vi "Check_Class_Spec.vi"(6 "ID String":string, 8 "error in (no error)":errorcluster, 9 "error out ref":refnum<vi>, 10 "vi refnum":refnum<vi>, 11 "ClassSpecifierConstant in":refnum<vi>) -> (0 "error out 2":errorcluster, 3 "OK":bool)   [LabVIEW 2025]
panel:
  out "error out":errorcluster
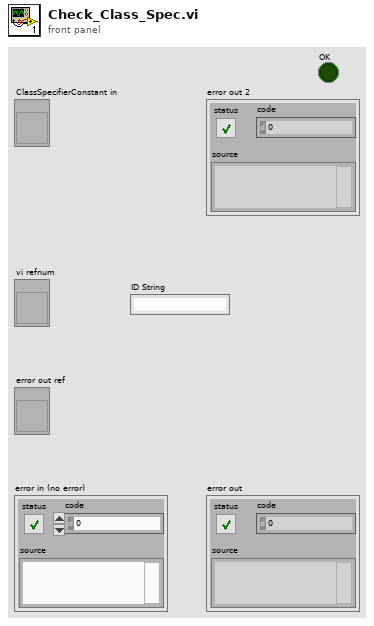
[diagram p1: front panel]
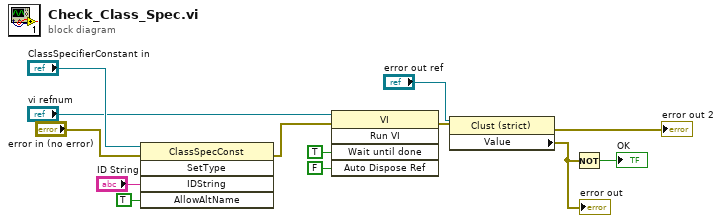
[diagram p0: block diagram]
diagram:
  n1 = invoke class="ClassSpecConst" method="SetType"(reference="ClassSpecifierConstant in", error in="error in (no error)", "IDString"="ID String", "AllowAltName"=TRUE ("Allow Alternate Name? (F)")) -> (error out=w11:errorcluster)  [unwired: 1 in, 4 out]
  n2 = invoke class="VI" method="Run VI"(reference="vi refnum", error in=w11, "Wait until done"=TRUE ("Wait Until Done"), "Auto Dispose Ref"=FALSE ("Auto Dispose Reference")) -> (error out=w6:errorcluster)  [unwired: 1 in, 4 out]
  n3 = property class="Clust (strict)"(reference="error out ref", error in=w6) -> (error out=→"error out 2":errorcluster, "Value"=w13:errorcluster)  [unwired: 1 out]
  "error out" <- w13
  n4 = Not(x=w13) -> (.not. x?=→"OK":bool)
